vi "Map LED Matrix.vi"(10 "length":i32=6, 11 "Image":bool[][](array[boolean])) -> (3 "Image - Mapped":bool[][](array[boolean]))   [LabVIEW 2017]
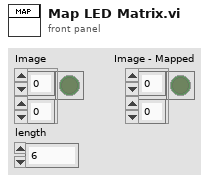
[diagram p1: front panel]
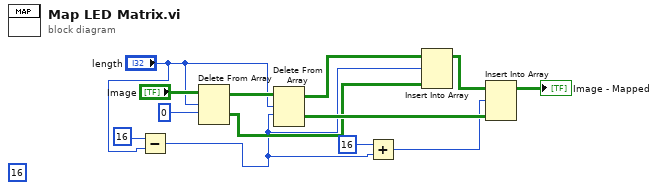
[diagram p0: block diagram]
diagram:
  (unwired) 16 ("x")
  n1 = Subtract(x=16, y="length") -> (x-y=w1:i32)
  n2 = Delete From Array(array="Image", length="length", index (row)=0) -> (deleted portion=w11:bool[][], array with subset deleted=w10:bool[][])  [unwired: 1 in]
  n3 = Delete From Array(array=w10, length="length", index (row)=w1) -> (deleted portion=w13:bool[][], array with subset deleted=w7:bool[][])  [unwired: 1 in]
  n4 = Add(x=16, y=w1) -> (x+y=w4:i32)
  n5 = Insert Into Array(array=w7, index (row)=w1, new element=w11) -> (w12:bool[][])  [unwired: 1 in]
  n6 = Insert Into Array(array=w12, index (row)=w4, new element=w13) -> (→"Image - Mapped":bool[][])  [unwired: 1 in]
